vi "AlliGator Get-Set Data Information.vi"(6 "Get (F)/Set (T)":bool, 8 "error in (no error)":errorcluster, 11 "Data Information in":T1={"Gates to Skip"={"Start"=0, "End"=0}, "# Gates"=0, "Gate Step"=0, "Gate Duration"=0.0, "Gate Separation"=0.0, "Pile-up Correction"=FALSE, "Pixel Well Capacity"=0, "Define Gates to"=enum."Skip", "Gates to Keep"={"First"=0, "Last"=0}, "Laser Period"=0.0, "SYNC Period"=0.0, "Channel Name"=0, "Channel Arithmetic"=enum."None", "Background File Subtraction"=FALSE, "Background Scaling Factor"=1.0, "Background File"=path "", "Background Pile-up Correction"=FALSE, "Background Pixel Well Capacity"=1, "Dataset Scaling Factor"=1.0} {"Background Pixel Well Capacity" min=1 step=1; "Channel Name" items=["Bottom INT Gate", "Bottom G2 Gate"]; "SYNC Period" min=0.0 format="%#.3g"; "Laser Period" min=0.0 format="%#.3g"; "Pixel Well Capacity" min=1 step=1; "# Gates" min=1 step=1; "Gate Step" min=1 step=1; "Gate Duration" min=1e-09 max=4.294967295 step=1e-09; "Gate Separation" min=0.0 format="%#.3g"}) -> (0 "error out":errorcluster, 3 "Data Information out":T1={"Gates to Skip"={"Start"=0, "End"=0}, "# Gates"=0, "Gate Step"=0, "Gate Duration"=0.0, "Gate Separation"=0.0, "Pile-up Correction"=FALSE, "Pixel Well Capacity"=0, "Define Gates to"=enum."Skip", "Gates to Keep"={"First"=0, "Last"=0}, "Laser Period"=0.0, "SYNC Period"=0.0, "Channel Name"=0, "Channel Arithmetic"=enum."None", "Background File Subtraction"=FALSE, "Background Scaling Factor"=1.0, "Background File"=path "", "Background Pile-up Correction"=FALSE, "Background Pixel Well Capacity"=1, "Dataset Scaling Factor"=1.0} {"Background Pixel Well Capacity" min=1 step=1; "Channel Name" items=["Bottom INT Gate", "Bottom G2 Gate"]; "SYNC Period" min=0.0 format="%#.3g"; "Laser Period" min=0.0 format="%#.3g"; "Pixel Well Capacity" min=1 step=1; "# Gates" min=1 step=1; "Gate Step" min=1 step=1; "Gate Duration" min=0.0 format="%#.3g"; "Gate Separation" min=0.0 format="%#.3g"})   [LabVIEW 2021, in "AlliGator Scripts.lvlib"]
doc: "Gets/Sets Dataset Information stored in the Settings Storage.vi"
uses:
  AlliGator Scripts.lvlib
  AlliGator Data Information.ctl
  Settings/AlliGator Background Subtraction Parameters.ctl
  Settings/AlliGator Define Gates to.ctl
  Settings/AlliGator Gates to Keep.ctl
  Settings/AlliGator Gate Arithmetic.ctl
  Settings/AlliGator Settings List.ctl
  Settings/AlliGator Settings.lvlib
panel:
  # "see the AlliGator License on the block diagram (Ctrl+E or Window:Show Block Diagram)"
  # "Gates Characteristics"
  # "Background File Subtraction"
  # "Gates Characteristics"
  # "Background File Subtraction"
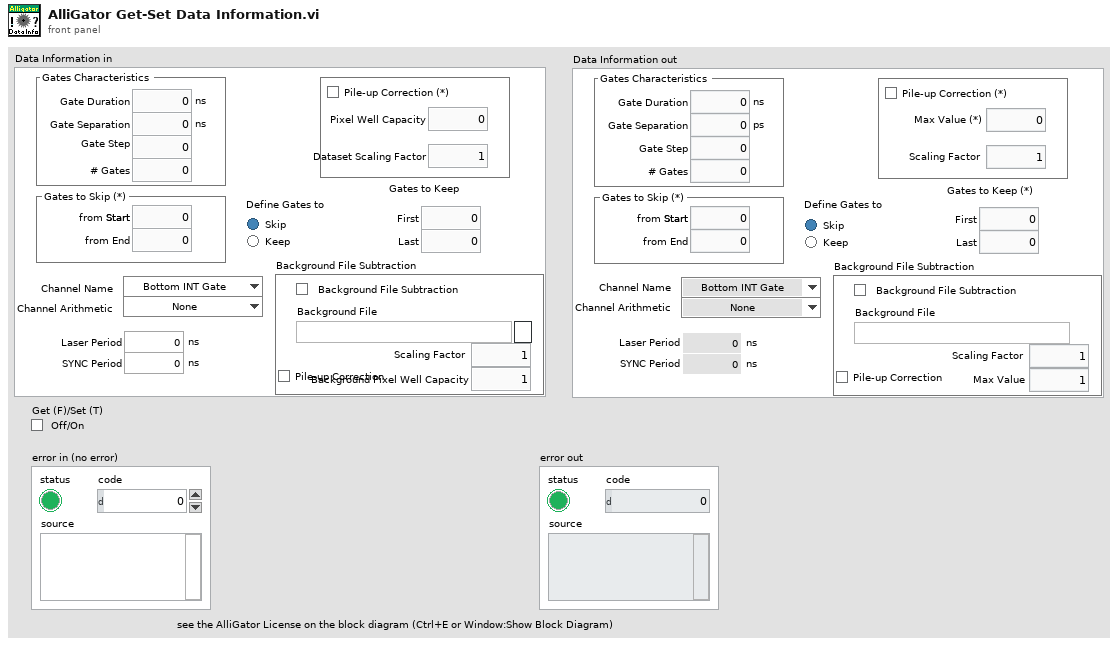
[diagram p1: front panel]
types:
  T1 = typedef "AlliGator Scripts.lvlib/AlliGator Data Information.ctl" = cluster{"Gates to Skip":T2, "# Gates":u32, "Gate Step":u32, "Gate Duration":dbl[unit], "Gate Separation":dbl[unit], "Pile-up Correction":bool, "Pixel Well Capacity":u32, "Define Gates to":T3, "Gates to Keep":T4, "Laser Period":dbl[unit], "SYNC Period":dbl[unit], "Channel Name":u16, "Channel Arithmetic":T5, "Background File Subtraction":bool, "Background Scaling Factor":dbl, "Background File":path, "Background Pile-up Correction":bool, "Background Pixel Well Capacity":u32, "Dataset Scaling Factor":dbl}
  T2 = typedef "AlliGator Settings.lvlib/AlliGator Background Subtraction Parameters.ctl" = cluster{"Start":u32, "End":u32}
  T3 = typedef "AlliGator Settings.lvlib/AlliGator Define Gates to.ctl" = enum32{"Skip", "Keep"}
  T4 = typedef "AlliGator Settings.lvlib/AlliGator Gates to Keep.ctl" = cluster{"First":u32, "Last":u32}
  T5 = typedef "AlliGator Settings.lvlib/AlliGator Gate Arithmetic.ctl" = enum16{"None", "INT-G2", "G2/INT*<INT>", "(1 - G2/INT)*<INT>"}
  T6 = typedef "AlliGator Settings.lvlib/AlliGator Settings List.ctl" = enum16{"GUI:Visible Settings Tab", "GUI:Last Run Version", "Source Image:Use Image Histogram for Contrast", "Source Image:Low Count Pixels Rejection Options", "Source Image:High Count Pixels Rejection Options", "Source Image:Use Image Brightness", "Source Image:Blend Overlay with Image Background", "Source Image:Use Fixed ROI Diameter", "Source Image:ROI Diameter", "Source Image:ROI Center Color", "Source Image:Peak Threshold", "Source Image:Intensity Threshold", "Source Image:Image Binning Options", "Source Image:Image Smoothing Options", "Source Image:Image Histogram Active", "Source Image:Invert Binary Mask", "Source Image:Hot Pixel Removal", "Source Image:Overlay Analyzed ROI Center", "Source Image:Auto-Adjust Contrast", "Source Image:Histogram Lower Percentile", "Source Image:Histogram Upper Percentile", "Source Image:Save Source Image", "Source Image:Scale Bar Options", "Source Image:Image Resolution (Pixel Size)", "Source Image:Flatfield Correction", "Source Image:Show Dead Left Columns Correction", "Source Image:Dead Left Columns Correction", "Source Image:Image Pre-Processing Operations Order", "Source Image:Overlay ROI Median", "Source Image:Median Overlay Color", "Data Information:Gate Width", "Data Information:Nanotime Gate Separation", "Data Information:Macrotime Gate Separation", "Data Information:Gate Step", "Data Information:# Gates", "Data Information:Gate Image Exposure", "Data Information:Gate Image Integration", "Data Information:Gates to Skip", "Data Information:Gates to Keep", "Data Information:Define Gates to", "Data Information:Channel Name", "Data Information:Available Channel Names", "Data Information:Channel Arithmetic", "Data Information:Background File Subtraction", "Data Information:Background File", "Data Information:Background Scaling Factor", "Data Information:Background Pile-up Correction", "Data Information:Background Pixel Well Capacity", "Data Information:Laser Period", "Data Information:SYNC Period", "Data Information:Pile-up Correction", "Data Information:Pixel Well Capacity", "Data Information:Dataset Scaling Factor", "Fluorescence Decay_Decay Pre-Processing:Reverse Gates", "Fluorescence Decay_Decay Pre-Processing:Verbose Decay Pre-Processing", "Fluorescence Decay_Decay Pre-Processing:Use Decay Pre-Processing", "Fluorescence Decay_Decay Pre-Processing:Background Subtraction", "Fluorescence Decay_Decay Pre-Processing:Background Definition Range", "Fluorescence Decay_Decay Pre-Processing:Baseline Subtraction Method", "Fluorescence Decay_Decay Pre-Processing:Decay Pre-Processing Operations Order", "Fluorescence Decay_Decay Pre-Processing:Smoothing Parameter", "Fluorescence Decay_Decay Pre-Processing:Shift Decay", "Fluorescence Decay_Decay Pre-Processing:Decay Shift Parameters", "Fluorescence Decay_Decay Pre-Processing:Fold Decay", "Fluorescence Decay_Decay Pre-Processing:# Folds", "Fluorescence Decay_Decay Pre-Processing:1-Normalize Decay", "Fluorescence Decay_Decay Pre-Processing:[0-1]-Normalize Decay", "Fluorescence Decay_Decay Pre-Processing:Smoothen Decay", "Fluorescence Decay_Decay Pre-Processing:Extrapolate Decay", "Fluorescence Decay_Decay Pre-Processing:Use Periodicity", "Fluorescence Decay_Decay Pre-Processing:Use Cursors", "Fluorescence Decay_Decay Pre-Processing:Tail Fraction", "Fluorescence Decay_Decay Pre-Processing:Head Fraction", "Fluorescence Decay_Decay Pre-Processing:Additional Points", "Fluorescence Decay_Decay Pre-Processing:Straighten Decay", "Fluorescence Decay_Decay Pre-Processing:Constant Background", "Fluorescence Decay_Decay Pre-Processing:Pixel-Normalize Decay", "Fluorescence Decay_Advanced Analysis:Extract IRF instead of Decay", "Fluorescence Decay_Advanced Analysis:IRF Extraction Options", "Fluorescence Decay_Advanced Analysis:IRF Optimization Options", "Fluorescence Decay_Advanced Analysis:Square Pulse Options", "Fluorescence Decay_Advanced Analysis:IRF Order", "Fluorescence Decay_Advanced Analysis:IRF Time Constants", "Fluorescence Decay_Advanced Analysis:Wavelet Analysis Options", "Fluorescence Decay_Advanced Analysis:Average Lifetime Options", "Fluorescence Decay_Fit Options:Fit Options", "Fluorescence Decay_Fit Options:Use Legacy Fitting Approach", "Fluorescence Decay_Fit Options:Use Data Information Laser Period", "Fluorescence Decay_Fit Parameters:Displayed Fit Parameters", "Fluorescence Decay_Fit Parameters:Fit Parameter Constraints", "Fluorescence Decay_Fit Parameters:Export Tabulated Results", "Fluorescence Decay_Fit Parameters:MLE Baseline Offset Type", "Fluorescence Decay_Fit Parameters:MLE Baseline Offset", "Fluorescence Decay_Fit Parameters:Guess Parameter Names", "Fluorescence Decay_Fit Parameters:Guess Parameter Values", "Fluorescence Decay_Fit Parameters:Guess Parameters Options", "Fluorescence Decay_Styles:Show Last Decay Only", "Fluorescence Decay_Styles:Decay Graph Color Array", "Fluorescence Decay:Decay Graph Active", "Fluorescence Decay Statistics:Min Peak Value", "Fluorescence Decay Statistics:Reject Low Decay Peak Pixels", "Fluorescence Decay Statistics:Reject High Decay Peak Pixels", "Fluorescence Decay Statistics:Max Peak Value", "Time Traces:Use File Timestamp", "Time Traces:Time Step", "Time Traces:Use Intensity Correction File", "Time Traces:Intensity Correction File", "Phasor Plot:Phasor Plot Smoothing Options", "Phasor Plot:Phasor Plot Size", "Phasor Plot:Phasor Plot Graphics Options", "Phasor Plot:Cumulative Phasor Plot", "Phasor Plot:Use Phasor Brightness", "Phasor Plot:Blend Overlay with Phasor Background", "Phasor Plot:Save Phasor Plot", "Phasor Plot:Show References", "Phasor Plot:Phasor Ratio Decay Range", "Phasor Plot:Exponential Fading", "Phasor Plot:Phasor Ratio Reference Colors", "Phasor Plot:Reference Radius", "Phasor Plot:Show Color Map Vertices", "Phasor Plot:Phasor Plot Active", "Phasor Plot:Phasor Ratio Color Map Type", "Phasor Plot:Phasor Ratio Color Map", "Phasor Plot:Phasor Ratio Display Range", "Phasor Plot:Selected Image ROI(s)", "Phasor Plot:All Image ROIs", "Phasor Plot:Selected Phasor Plot ROI(s)", "Phasor Plot:All Phasor Plot ROIs", "Phasor Plot:Phasor Ratio Color-Coded Quantity", "Phasor Plot:Store Phasor Harmonics", "Phasor Plot:Draw Reference Segment", "Phasor Plot:User-Defined Quantity", "Phasor Graph:Phasor Frequency", "Phasor Graph:Phasor Ratio Type", "Phasor Graph:Pixel-level Phasor Computation", "Phasor Graph:Save Phasor Graph", "Phasor Graph:Phasor Graph Active", "Phasor Graph:Phasor SDV Options", "Phasor Calibration:Use Backup Calibration if needed", "Phasor Graph:Define Shortest Lifetime as", "Phasor Calibration:Backup Calibration Type", "Phasor Calibration:Calibration Type", "Phasor Calibration:Calibration Lifetime", "Phasor Calibration:Calibration Map Algorithm", "Single-Exponential Phasor Locus (SEPL):Gate Parameters", "Single-Exponential Phasor Locus (SEPL):User-defined Gate", "Single-Exponential Phasor Locus (SEPL):User-defined IRF", "Single-Exponential Phasor Locus (SEPL):Phasor Parameters", "Single-Exponential Phasor Locus (SEPL):Decay & IRF Parameters", "Single-Exponential Phasor Locus (SEPL):Display Parameters", "Lifetime Analysis:Decay Analysis Parameters", "Lifetime Analysis:Lifetime Map Active", "Plugins:Python Settings", "Miscellaneous:Verbose Mode", "Miscellaneous:Beep after Script", "Miscellaneous:Saved Image File Format", "Miscellaneous:Exported Gate Image Settings", "Miscellaneous:Include Loading in Timing", "Miscellaneous:Verbose Settings Mode", "Miscellaneous:Histogram Options", "Miscellaneous:Beep on Error", "Miscellaneous:# Logical Processors Used", "Miscellaneous:ROI Description Max Characters", "Miscellaneous:Verbose Error Mode", "Miscellaneous:Transparent Mask Color"}
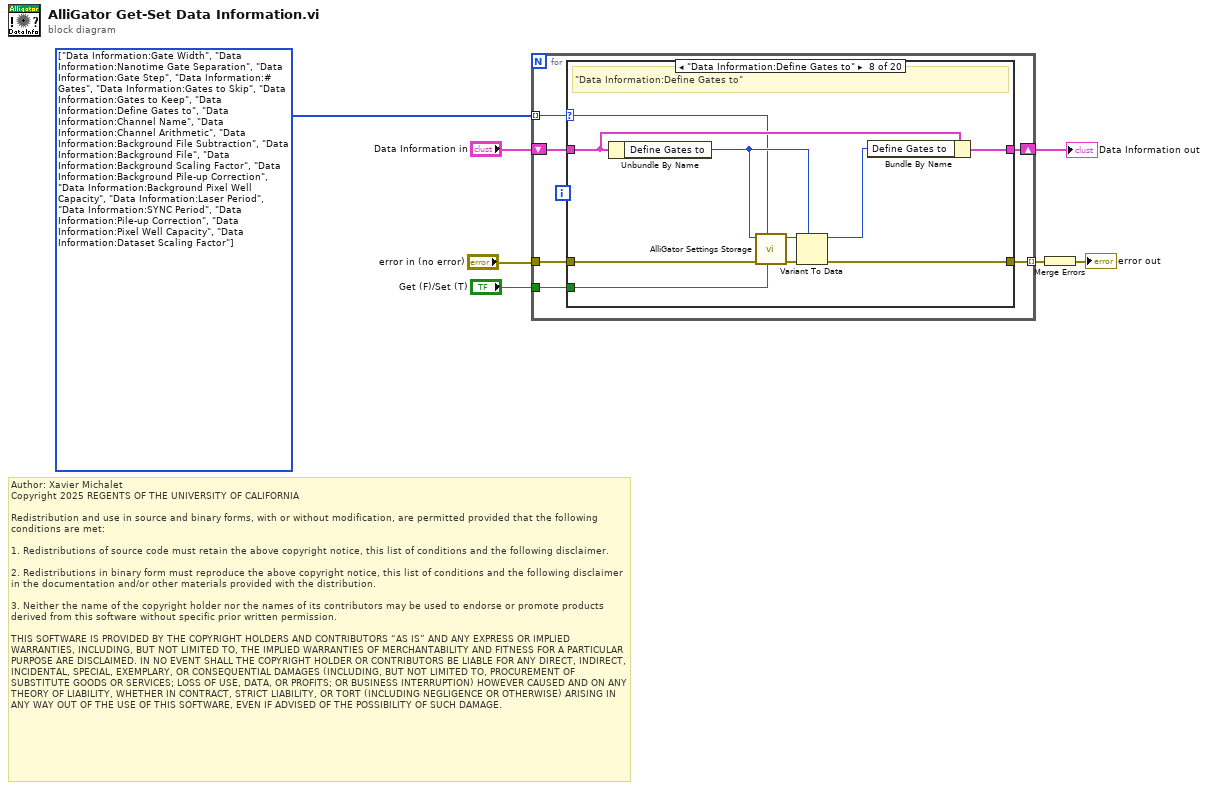
[diagram p0: block diagram]
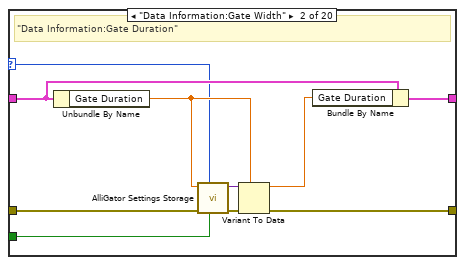
[diagram p3: hidden frame]
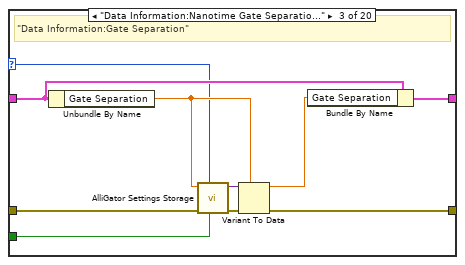
[diagram p4: hidden frame]
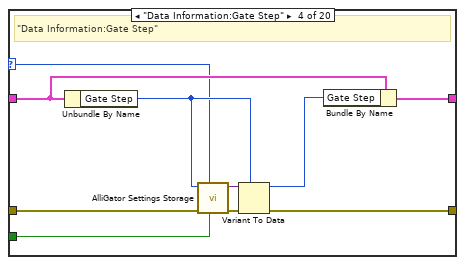
[diagram p5: hidden frame]
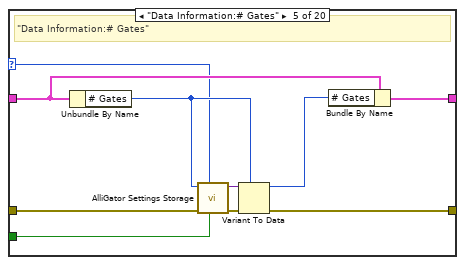
[diagram p6: hidden frame]
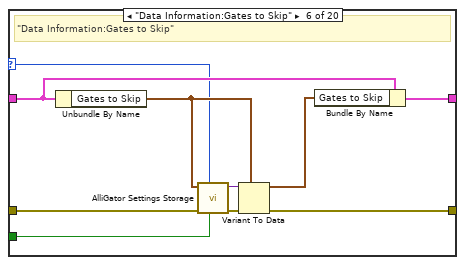
[diagram p7: hidden frame]
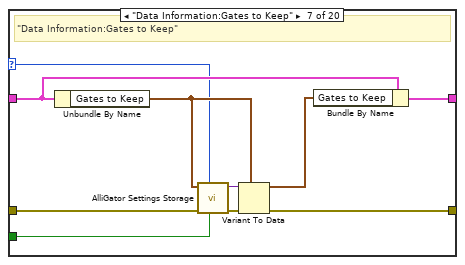
[diagram p8: hidden frame]
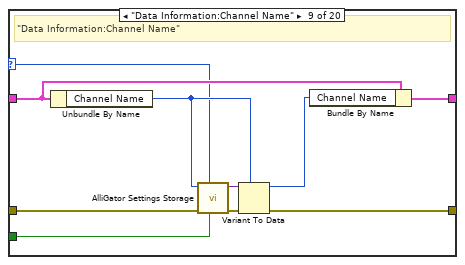
[diagram p9: hidden frame]
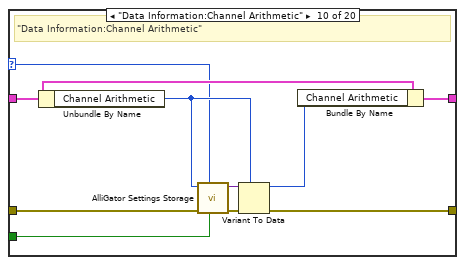
[diagram p10: hidden frame]
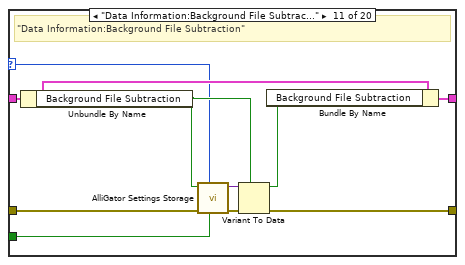
[diagram p11: hidden frame]
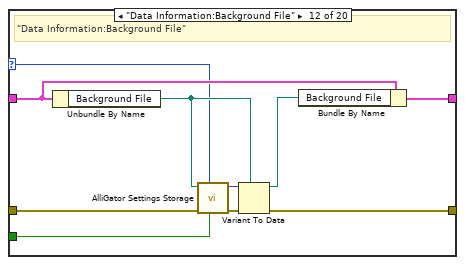
[diagram p12: hidden frame]
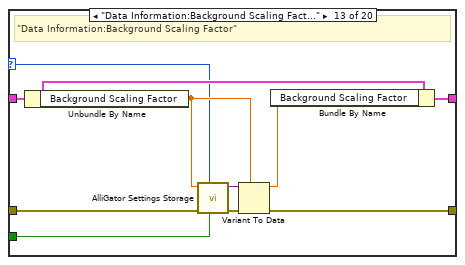
[diagram p13: hidden frame]
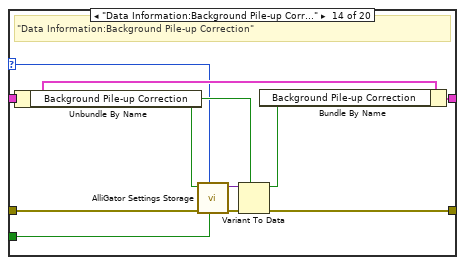
[diagram p14: hidden frame]
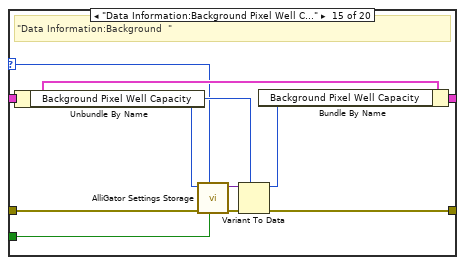
[diagram p15: hidden frame]
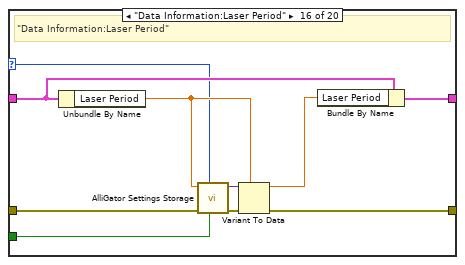
[diagram p16: hidden frame]
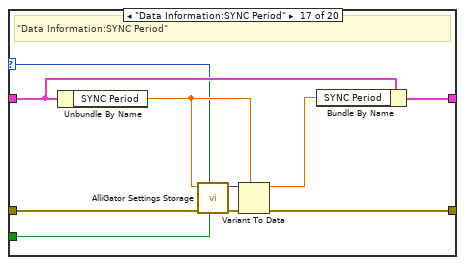
[diagram p17: hidden frame]
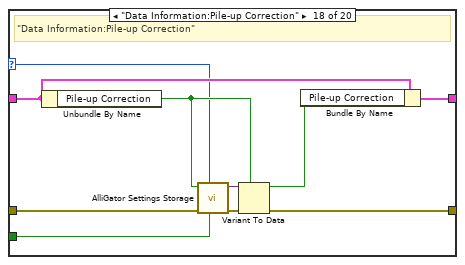
[diagram p18: hidden frame]
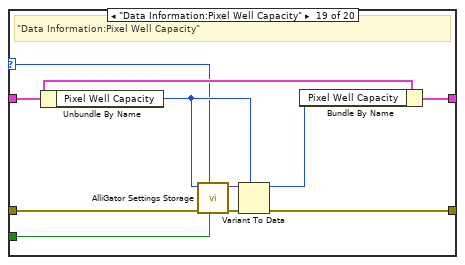
[diagram p19: hidden frame]
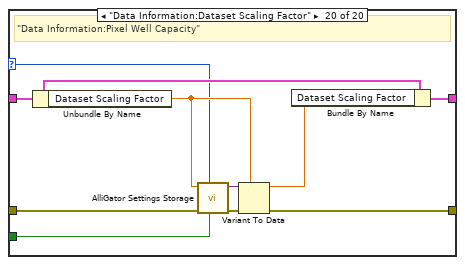
[diagram p20: hidden frame]
diagram:
  w1 = T6[] [enum."Data Information:Gate Width", enum."Data Information:Nanotime Gate Separation", enum."Data Information:Gate Step", enum."Data Information:# Gates", enum."Data Information:Gates to Skip", enum."Data Information:Gates to Keep", enum."Data Information:Define Gates to", enum."Data Information:Channel Name", enum."Data Information:Channel Arithmetic", enum."Data Information:Background File Subtraction", enum."Data Information:Background File", enum."Data Information:Background Scaling Factor", enum."Data Information:Background Pile-up Correction", enum."Data Information:Background Pixel Well Capacity", enum."Data Information:Laser Period", enum."Data Information:SYNC Period", enum."Data Information:Pile-up Correction", enum."Data Information:Pixel Well Capacity", enum."Data Information:Dataset Scaling Factor"] items=["GUI:Visible Settings Tab", "GUI:Last Run Version", "Source Image:Use Image Histogram for Contrast", "Source Image:Low Count Pixels Rejection Options", "Source Image:High Count Pixels Rejection Options", "Source Image:Use Image Brightness", "Source Image:Blend Overlay with Image Background", "Source Image:Use Fixed ROI Diameter", "Source Image:ROI Diameter", "Source Image:ROI Center Color", "Source Image:Peak Threshold", "Source Image:Intensity Threshold", "Source Image:Image Binning Options", "Source Image:Image Smoothing Options", "Source Image:Image Histogram Active", "Source Image:Invert Binary Mask", "Source Image:Hot Pixel Removal", "Source Image:Overlay Analyzed ROI Center", "Source Image:Auto-Adjust Contrast", "Source Image:Histogram Lower Percentile", "Source Image:Histogram Upper Percentile", "Source Image:Save Source Image", "Source Image:Scale Bar Options", "Source Image:Image Resolution (Pixel Size)", "Source Image:Flatfield Correction", "Source Image:Show Dead Left Columns Correction", "Source Image:Dead Left Columns Correction", "Source Image:Image Pre-Processing Operations Order", "Source Image:Overlay ROI Median", "Source Image:Median Overlay Color", "Data Information:Gate Width", "Data Information:Nanotime Gate Separation", "Data Information:Macrotime Gate Separation", "Data Information:Gate Step", "Data Information:# Gates", "Data Information:Gate Image Exposure", "Data Information:Gate Image Integration", "Data Information:Gates to Skip", "Data Information:Gates to Keep", "Data Information:Define Gates to", "Data Information:Channel Name", "Data Information:Available Channel Names", "Data Information:Channel Arithmetic", "Data Information:Background File Subtraction", "Data Information:Background File", "Data Information:Background Scaling Factor", "Data Information:Background Pile-up Correction", "Data Information:Background Pixel Well Capacity", "Data Information:Laser Period", "Data Information:SYNC Period", "Data Information:Pile-up Correction", "Data Information:Pixel Well Capacity", "Data Information:Dataset Scaling Factor", "Fluorescence Decay_Decay Pre-Processing:Reverse Gates", "Fluorescence Decay_Decay Pre-Processing:Verbose Decay Pre-Processing", "Fluorescence Decay_Decay Pre-Processing:Use Decay Pre-Processing", "Fluorescence Decay_Decay Pre-Processing:Background Subtraction", "Fluorescence Decay_Decay Pre-Processing:Background Definition Range", "Fluorescence Decay_Decay Pre-Processing:Baseline Subtraction Method", "Fluorescence Decay_Decay Pre-Processing:Decay Pre-Processing Operations Order", "Fluorescence Decay_Decay Pre-Processing:Smoothing Parameter", "Fluorescence Decay_Decay Pre-Processing:Shift Decay", "Fluorescence Decay_Decay Pre-Processing:Decay Shift Parameters", "Fluorescence Decay_Decay Pre-Processing:Fold Decay", "Fluorescence Decay_Decay Pre-Processing:# Folds", "Fluorescence Decay_Decay Pre-Processing:1-Normalize Decay", "Fluorescence Decay_Decay Pre-Processing:[0-1]-Normalize Decay", "Fluorescence Decay_Decay Pre-Processing:Smoothen Decay", "Fluorescence Decay_Decay Pre-Processing:Extrapolate Decay", "Fluorescence Decay_Decay Pre-Processing:Use Periodicity", "Fluorescence Decay_Decay Pre-Processing:Use Cursors", "Fluorescence Decay_Decay Pre-Processing:Tail Fraction", "Fluorescence Decay_Decay Pre-Processing:Head Fraction", "Fluorescence Decay_Decay Pre-Processing:Additional Points", "Fluorescence Decay_Decay Pre-Processing:Straighten Decay", "Fluorescence Decay_Decay Pre-Processing:Constant Background", "Fluorescence Decay_Decay Pre-Processing:Pixel-Normalize Decay", "Fluorescence Decay_Advanced Analysis:Extract IRF instead of Decay", "Fluorescence Decay_Advanced Analysis:IRF Extraction Options", "Fluorescence Decay_Advanced Analysis:IRF Optimization Options", "Fluorescence Decay_Advanced Analysis:Square Pulse Options", "Fluorescence Decay_Advanced Analysis:IRF Order", "Fluorescence Decay_Advanced Analysis:IRF Time Constants", "Fluorescence Decay_Advanced Analysis:Wavelet Analysis Options", "Fluorescence Decay_Advanced Analysis:Average Lifetime Options", "Fluorescence Decay_Fit Options:Fit Options", "Fluorescence Decay_Fit Options:Use Legacy Fitting Approach", "Fluorescence Decay_Fit Options:Use Data Information Laser Period", "Fluorescence Decay_Fit Parameters:Displayed Fit Parameters", "Fluorescence Decay_Fit Parameters:Fit Parameter Constraints", "Fluorescence Decay_Fit Parameters:Export Tabulated Results", "Fluorescence Decay_Fit Parameters:MLE Baseline Offset Type", "Fluorescence Decay_Fit Parameters:MLE Baseline Offset", "Fluorescence Decay_Fit Parameters:Guess Parameter Names", "Fluorescence Decay_Fit Parameters:Guess Parameter Values", "Fluorescence Decay_Fit Parameters:Guess Parameters Options", "Fluorescence Decay_Styles:Show Last Decay Only", "Fluorescence Decay_Styles:Decay Graph Color Array", "Fluorescence Decay:Decay Graph Active", "Fluorescence Decay Statistics:Min Peak Value", "Fluorescence Decay Statistics:Reject Low Decay Peak Pixels", "Fluorescence Decay Statistics:Reject High Decay Peak Pixels", "Fluorescence Decay Statistics:Max Peak Value", "Time Traces:Use File Timestamp", "Time Traces:Time Step", "Time Traces:Use Intensity Correction File", "Time Traces:Intensity Correction File", "Phasor Plot:Phasor Plot Smoothing Options", "Phasor Plot:Phasor Plot Size", "Phasor Plot:Phasor Plot Graphics Options", "Phasor Plot:Cumulative Phasor Plot", "Phasor Plot:Use Phasor Brightness", "Phasor Plot:Blend Overlay with Phasor Background", "Phasor Plot:Save Phasor Plot", "Phasor Plot:Show References", "Phasor Plot:Phasor Ratio Decay Range", "Phasor Plot:Exponential Fading", "Phasor Plot:Phasor Ratio Reference Colors", "Phasor Plot:Reference Radius", "Phasor Plot:Show Color Map Vertices", "Phasor Plot:Phasor Plot Active", "Phasor Plot:Phasor Ratio Color Map Type", "Phasor Plot:Phasor Ratio Color Map", "Phasor Plot:Phasor Ratio Display Range", "Phasor Plot:Selected Image ROI(s)", "Phasor Plot:All Image ROIs", "Phasor Plot:Selected Phasor Plot ROI(s)", "Phasor Plot:All Phasor Plot ROIs", "Phasor Plot:Phasor Ratio Color-Coded Quantity", "Phasor Plot:Store Phasor Harmonics", "Phasor Plot:Draw Reference Segment", "Phasor Plot:User-Defined Quantity", "Phasor Graph:Phasor Frequency", "Phasor Graph:Phasor Ratio Type", "Phasor Graph:Pixel-level Phasor Computation", "Phasor Graph:Save Phasor Graph", "Phasor Graph:Phasor Graph Active", "Phasor Graph:Phasor SDV Options", "Phasor Calibration:Use Backup Calibration if needed", "Phasor Graph:Define Shortest Lifetime as", "Phasor Calibration:Backup Calibration Type", "Phasor Calibration:Calibration Type", "Phasor Calibration:Calibration Lifetime", "Phasor Calibration:Calibration Map Algorithm", "Single-Exponential Phasor Locus (SEPL):Gate Parameters", "Single-Exponential Phasor Locus (SEPL):User-defined Gate", "Single-Exponential Phasor Locus (SEPL):User-defined IRF", "Single-Exponential Phasor Locus (SEPL):Phasor Parameters", "Single-Exponential Phasor Locus (SEPL):Decay & IRF Parameters", "Single-Exponential Phasor Locus (SEPL):Display Parameters", "Lifetime Analysis:Decay Analysis Parameters", "Lifetime Analysis:Lifetime Map Active", "Plugins:Python Settings", "Miscellaneous:Verbose Mode", "Miscellaneous:Beep after Script", "Miscellaneous:Saved Image File Format", "Miscellaneous:Exported Gate Image Settings", "Miscellaneous:Include Loading in Timing", "Miscellaneous:Verbose Settings Mode", "Miscellaneous:Histogram Options", "Miscellaneous:Beep on Error", "Miscellaneous:# Logical Processors Used", "Miscellaneous:ROI Description Max Characters", "Miscellaneous:Verbose Error Mode", "Miscellaneous:Transparent Mask Color"] ("Array")
  # "Author: Xavier Michalet\nCopyright 2025 REGENTS OF THE UNIVERSITY OF CALIFORNIA\n\nRedistribution and use in source and binary forms, with or without modification, are permitted provided that the following conditions are met:\n\n1. Redistributions of source code must retain the above copyright notice, this list of conditions and the following disclaimer.\n\n2. Redistributions in binary form must reproduce the above copyright notice, this list of conditions and the following disclaimer in the documentation and/or other materials provided with the distribution.\n\n3. Neither the name of the copyright holder nor the names of its contributors may be used to endorse or promote products derived from this software without specific prior written permission.\n\nTHIS SOFTWARE IS PROVIDED BY THE COPYRIGHT HOLDERS AND CONTRIBUTORS “AS IS” AND ANY EXPRESS OR IMPLIED WARRANTIES, INCLUDING, BUT NOT LIMITED TO, THE IMPLIED WARRANTIES OF MERCHANTABILITY AND FITNESS FOR A PARTICULAR PURPOSE ARE DISCLAIMED. IN NO EVENT SHALL THE COPYRIGHT HOLDER OR CONTRIBUTORS BE LIABLE FOR ANY DIRECT, INDIRECT, INCIDENTAL, SPECIAL, EXEMPLARY, OR CONSEQUENTIAL DAMAGES (INCLUDING, BUT NOT LIMITED TO, PROCUREMENT OF SUBSTITUTE GOODS OR SERVICES; LOSS OF USE, DATA, OR PROFITS; OR BUSINESS INTERRUPTION) HOWEVER CAUSED AND ON ANY THEORY OF LIABILITY, WHETHER IN CONTRACT, STRICT LIABILITY, OR TORT (INCLUDING NEGLIGENCE OR OTHERWISE) ARISING IN ANY WAY OUT OF THE USE OF THIS SOFTWARE, EVEN IF ADVISED OF THE POSSIBILITY OF SUCH DAMAGE."
  n1 = for {
    tunnel: "Get (F)/Set (T)" -> [w13]
    shift-right: [w8] -> w4
    shift-left: "Data Information in" -> [w11]
    tunnel: "error in (no error)" -> [w12]
    tunnel: [w10] -> w3 mode=indexing
    tunnel: w1 -> [w9] mode=indexing
    n2 = case shown="\"Data Information:Define Gates to\"" w9 {
      selector: w9 -> [_ w16 w26 w36 w46 w56 w66 w76 w86 w96 w106 w116 w126 w136 w146 w156 w166 w176 w186 w196]
      tunnel: w13 -> [_ w25 w35 w45 w55 w65 w75 w85 w95 w105 w115 w125 w135 w145 w155 w165 w175 w185 w195 w205]
      tunnel: w12 -> [w14 w24 w34 w44 w54 w64 w74 w84 w94 w104 w114 w124 w134 w144 w154 w164 w174 w184 w194 w204]
      tunnel: w11 -> [w15 w18 w28 w38 w48 w58 w68 w78 w88 w98 w108 w118 w128 w138 w148 w158 w168 w178 w188 w198]
      tunnel: [w14 w17 w27 w37 w47 w57 w67 w77 w87 w97 w107 w117 w127 w137 w147 w157 w167 w177 w187 w197] -> w10
      tunnel: [w15 w19 w29 w39 w49 w59 w69 w79 w89 w99 w109 w119 w129 w139 w149 w159 w169 w179 w189 w199] -> w8
      frame "Miscellaneous:Verbose Mode", Default {
      }
      frame "Data Information:Gate Width" {
        # "\"Data Information:Gate Duration\""
        n3 = Unbundle By Name(w18) -> ("Gate Duration"=w20:dbl[unit])
        n4 = call "AlliGator Settings Storage.vi"("Get(F)/Set"=w25, "AlliGator Settings List"=w16, "Error In"=w24, "Variant Data in"=w20) -> ("Error Out"=w23:errorcluster, "Variant Data out"=w22:variant)  [unwired: 6 in]
        n5 = Variant To Data(error in=w23, type=w20, Variant=w22) -> (data=w21:dbl[unit], error out=w17:errorcluster)
        n6 = Bundle By Name(cluster=w18, "Gate Duration"=w21) -> (w19:T1)
      }
      frame "Data Information:Nanotime Gate Separation" {
        # "\"Data Information:Gate Separation\""
        n7 = Unbundle By Name(w28) -> ("Gate Separation"=w30:dbl[unit])
        n8 = call "AlliGator Settings Storage.vi"("Get(F)/Set"=w35, "AlliGator Settings List"=w26, "Error In"=w34, "Variant Data in"=w30) -> ("Error Out"=w33:errorcluster, "Variant Data out"=w32:variant)  [unwired: 6 in]
        n9 = Variant To Data(error in=w33, type=w30, Variant=w32) -> (data=w31:dbl[unit], error out=w27:errorcluster)
        n10 = Bundle By Name(cluster=w28, "Gate Separation"=w31) -> (w29:T1)
      }
      frame "Data Information:Gate Step" {
        # "\"Data Information:Gate Step\""
        n11 = Unbundle By Name(w38) -> ("Gate Step"=w40:u32)
        n12 = call "AlliGator Settings Storage.vi"("Get(F)/Set"=w45, "AlliGator Settings List"=w36, "Error In"=w44, "Variant Data in"=w40) -> ("Error Out"=w43:errorcluster, "Variant Data out"=w42:variant)  [unwired: 6 in]
        n13 = Variant To Data(error in=w43, type=w40, Variant=w42) -> (data=w41:u32, error out=w37:errorcluster)
        n14 = Bundle By Name(cluster=w38, "Gate Step"=w41) -> (w39:T1)
      }
      frame "Data Information:# Gates" {
        # "\"Data Information:# Gates\""
        n15 = Unbundle By Name(w48) -> ("# Gates"=w50:u32)
        n16 = call "AlliGator Settings Storage.vi"("Get(F)/Set"=w55, "AlliGator Settings List"=w46, "Error In"=w54, "Variant Data in"=w50) -> ("Error Out"=w53:errorcluster, "Variant Data out"=w52:variant)  [unwired: 6 in]
        n17 = Variant To Data(error in=w53, type=w50, Variant=w52) -> (data=w51:u32, error out=w47:errorcluster)
        n18 = Bundle By Name(cluster=w48, "# Gates"=w51) -> (w49:T1)
      }
      frame "Data Information:Gates to Skip" {
        # "\"Data Information:Gates to Skip\""
        n19 = Unbundle By Name(w58) -> ("Gates to Skip"=w60:T2)
        n20 = call "AlliGator Settings Storage.vi"("Get(F)/Set"=w65, "AlliGator Settings List"=w56, "Error In"=w64, "Variant Data in"=w60) -> ("Error Out"=w63:errorcluster, "Variant Data out"=w62:variant)  [unwired: 6 in]
        n21 = Variant To Data(error in=w63, type=w60, Variant=w62) -> (data=w61:T2, error out=w57:errorcluster)
        n22 = Bundle By Name(cluster=w58, "Gates to Skip"=w61) -> (w59:T1)
      }
      frame "Data Information:Gates to Keep" {
        # "\"Data Information:Gates to Keep\""
        n23 = Unbundle By Name(w68) -> ("Gates to Keep"=w70:T4)
        n24 = call "AlliGator Settings Storage.vi"("Get(F)/Set"=w75, "AlliGator Settings List"=w66, "Error In"=w74, "Variant Data in"=w70) -> ("Error Out"=w73:errorcluster, "Variant Data out"=w72:variant)  [unwired: 6 in]
        n25 = Variant To Data(error in=w73, type=w70, Variant=w72) -> (data=w71:T4, error out=w67:errorcluster)
        n26 = Bundle By Name(cluster=w68, "Gates to Keep"=w71) -> (w69:T1)
      }
      frame "Data Information:Define Gates to" {
        # "\"Data Information:Define Gates to\""
        n27 = Unbundle By Name(w78) -> ("Define Gates to"=w80:T3)
        n28 = call "AlliGator Settings Storage.vi"("Get(F)/Set"=w85, "AlliGator Settings List"=w76, "Error In"=w84, "Variant Data in"=w80) -> ("Error Out"=w83:errorcluster, "Variant Data out"=w82:variant)  [unwired: 6 in]
        n29 = Variant To Data(error in=w83, type=w80, Variant=w82) -> (data=w81:T3, error out=w77:errorcluster)
        n30 = Bundle By Name(cluster=w78, "Define Gates to"=w81) -> (w79:T1)
      }
      frame "Data Information:Channel Name" {
        # "\"Data Information:Channel Name\""
        n31 = Unbundle By Name(w88) -> ("Channel Name"=w90:u16)
        n32 = call "AlliGator Settings Storage.vi"("Get(F)/Set"=w95, "AlliGator Settings List"=w86, "Error In"=w94, "Variant Data in"=w90) -> ("Error Out"=w93:errorcluster, "Variant Data out"=w92:variant)  [unwired: 6 in]
        n33 = Variant To Data(error in=w93, type=w90, Variant=w92) -> (data=w91:u16, error out=w87:errorcluster)
        n34 = Bundle By Name(cluster=w88, "Channel Name"=w91) -> (w89:T1)
      }
      frame "Data Information:Channel Arithmetic" {
        # "\"Data Information:Channel Arithmetic\""
        n35 = Unbundle By Name(w98) -> ("Channel Arithmetic"=w100:T5)
        n36 = call "AlliGator Settings Storage.vi"("Get(F)/Set"=w105, "AlliGator Settings List"=w96, "Error In"=w104, "Variant Data in"=w100) -> ("Error Out"=w103:errorcluster, "Variant Data out"=w102:variant)  [unwired: 6 in]
        n37 = Variant To Data(error in=w103, type=w100, Variant=w102) -> (data=w101:T5, error out=w97:errorcluster)
        n38 = Bundle By Name(cluster=w98, "Channel Arithmetic"=w101) -> (w99:T1)
      }
      frame "Data Information:Background File Subtraction" {
        # "\"Data Information:Background File Subtraction\""
        n39 = Unbundle By Name(w108) -> ("Background File Subtraction"=w110:bool)
        n40 = call "AlliGator Settings Storage.vi"("Get(F)/Set"=w115, "AlliGator Settings List"=w106, "Error In"=w114, "Variant Data in"=w110) -> ("Error Out"=w113:errorcluster, "Variant Data out"=w112:variant)  [unwired: 6 in]
        n41 = Variant To Data(error in=w113, type=w110, Variant=w112) -> (data=w111:bool, error out=w107:errorcluster)
        n42 = Bundle By Name(cluster=w108, "Background File Subtraction"=w111) -> (w109:T1)
      }
      frame "Data Information:Background File" {
        # "\"Data Information:Background File\""
        n43 = Unbundle By Name(w118) -> ("Background File"=w120:path)
        n44 = call "AlliGator Settings Storage.vi"("Get(F)/Set"=w125, "AlliGator Settings List"=w116, "Error In"=w124, "Variant Data in"=w120) -> ("Error Out"=w123:errorcluster, "Variant Data out"=w122:variant)  [unwired: 6 in]
        n45 = Variant To Data(error in=w123, type=w120, Variant=w122) -> (data=w121:path, error out=w117:errorcluster)
        n46 = Bundle By Name(cluster=w118, "Background File"=w121) -> (w119:T1)
      }
      frame "Data Information:Background Scaling Factor" {
        # "\"Data Information:Background Scaling Factor\""
        n47 = Unbundle By Name(w128) -> ("Background Scaling Factor"=w130:dbl)
        n48 = call "AlliGator Settings Storage.vi"("Get(F)/Set"=w135, "AlliGator Settings List"=w126, "Error In"=w134, "Variant Data in"=w130) -> ("Error Out"=w133:errorcluster, "Variant Data out"=w132:variant)  [unwired: 6 in]
        n49 = Variant To Data(error in=w133, type=w130, Variant=w132) -> (data=w131:dbl, error out=w127:errorcluster)
        n50 = Bundle By Name(cluster=w128, "Background Scaling Factor"=w131) -> (w129:T1)
      }
      frame "Data Information:Background Pile-up Correction" {
        # "\"Data Information:Background Pile-up Correction\""
        n51 = Unbundle By Name(w138) -> ("Background Pile-up Correction"=w140:bool)
        n52 = call "AlliGator Settings Storage.vi"("Get(F)/Set"=w145, "AlliGator Settings List"=w136, "Error In"=w144, "Variant Data in"=w140) -> ("Error Out"=w143:errorcluster, "Variant Data out"=w142:variant)  [unwired: 6 in]
        n53 = Variant To Data(error in=w143, type=w140, Variant=w142) -> (data=w141:bool, error out=w137:errorcluster)
        n54 = Bundle By Name(cluster=w138, "Background Pile-up Correction"=w141) -> (w139:T1)
      }
      frame "Data Information:Background Pixel Well Capacity" {
        # "\"Data Information:Background  \""
        n55 = Unbundle By Name(w148) -> ("Background Pixel Well Capacity"=w150:u32)
        n56 = call "AlliGator Settings Storage.vi"("Get(F)/Set"=w155, "AlliGator Settings List"=w146, "Error In"=w154, "Variant Data in"=w150) -> ("Error Out"=w153:errorcluster, "Variant Data out"=w152:variant)  [unwired: 6 in]
        n57 = Variant To Data(error in=w153, type=w150, Variant=w152) -> (data=w151:u32, error out=w147:errorcluster)
        n58 = Bundle By Name(cluster=w148, "Background Pixel Well Capacity"=w151) -> (w149:T1)
      }
      frame "Data Information:Laser Period" {
        # "\"Data Information:Laser Period\""
        n59 = Unbundle By Name(w158) -> ("Laser Period"=w160:dbl[unit])
        n60 = call "AlliGator Settings Storage.vi"("Get(F)/Set"=w165, "AlliGator Settings List"=w156, "Error In"=w164, "Variant Data in"=w160) -> ("Error Out"=w163:errorcluster, "Variant Data out"=w162:variant)  [unwired: 6 in]
        n61 = Variant To Data(error in=w163, type=w160, Variant=w162) -> (data=w161:dbl[unit], error out=w157:errorcluster)
        n62 = Bundle By Name(cluster=w158, "Laser Period"=w161) -> (w159:T1)
      }
      frame "Data Information:SYNC Period" {
        # "\"Data Information:SYNC Period\""
        n63 = Unbundle By Name(w168) -> ("SYNC Period"=w170:dbl[unit])
        n64 = call "AlliGator Settings Storage.vi"("Get(F)/Set"=w175, "AlliGator Settings List"=w166, "Error In"=w174, "Variant Data in"=w170) -> ("Error Out"=w173:errorcluster, "Variant Data out"=w172:variant)  [unwired: 6 in]
        n65 = Variant To Data(error in=w173, type=w170, Variant=w172) -> (data=w171:dbl[unit], error out=w167:errorcluster)
        n66 = Bundle By Name(cluster=w168, "SYNC Period"=w171) -> (w169:T1)
      }
      frame "Data Information:Pile-up Correction" {
        # "\"Data Information:Pile-up Correction\""
        n67 = Unbundle By Name(w178) -> ("Pile-up Correction"=w180:bool)
        n68 = call "AlliGator Settings Storage.vi"("Get(F)/Set"=w185, "AlliGator Settings List"=w176, "Error In"=w184, "Variant Data in"=w180) -> ("Error Out"=w183:errorcluster, "Variant Data out"=w182:variant)  [unwired: 6 in]
        n69 = Variant To Data(error in=w183, type=w180, Variant=w182) -> (data=w181:bool, error out=w177:errorcluster)
        n70 = Bundle By Name(cluster=w178, "Pile-up Correction"=w181) -> (w179:T1)
      }
      frame "Data Information:Pixel Well Capacity" {
        # "\"Data Information:Pixel Well Capacity\""
        n71 = Unbundle By Name(w188) -> ("Pixel Well Capacity"=w190:u32)
        n72 = call "AlliGator Settings Storage.vi"("Get(F)/Set"=w195, "AlliGator Settings List"=w186, "Error In"=w194, "Variant Data in"=w190) -> ("Error Out"=w193:errorcluster, "Variant Data out"=w192:variant)  [unwired: 6 in]
        n73 = Variant To Data(error in=w193, type=w190, Variant=w192) -> (data=w191:u32, error out=w187:errorcluster)
        n74 = Bundle By Name(cluster=w188, "Pixel Well Capacity"=w191) -> (w189:T1)
      }
      frame "Data Information:Dataset Scaling Factor" {
        # "\"Data Information:Pixel Well Capacity\""
        n75 = Unbundle By Name(w198) -> ("Dataset Scaling Factor"=w200:dbl)
        n76 = call "AlliGator Settings Storage.vi"("Get(F)/Set"=w205, "AlliGator Settings List"=w196, "Error In"=w204, "Variant Data in"=w200) -> ("Error Out"=w203:errorcluster, "Variant Data out"=w202:variant)  [unwired: 6 in]
        n77 = Variant To Data(error in=w203, type=w200, Variant=w202) -> (data=w201:dbl, error out=w197:errorcluster)
        n78 = Bundle By Name(cluster=w198, "Dataset Scaling Factor"=w201) -> (w199:T1)
      }
    }
  }
  "Data Information out" <- w4
  n79 = Merge Errors(w3) -> (→"error out":errorcluster)
